vi "更新程序.vi"() -> ()   [LabVIEW 2016, in "自动更新.lvlib"]
uses:
  <vilib>/FTP/NI_FTP.lvlib
panel:
  out "updateconfiguration":T1
  out "软件版本 2":string caption="目标软件版本"
  out "软件版本":string caption="当前软件版本"
  out "下载的文件名":string
  out "目标文件夹名":string
  out "端口号":i32
  out "IP地址":string
  out "步骤":string
  out "枚举":T2(ring)
  in  "目标路径（使用对话框）":path
  out "下载保存目录":path
  out "更新进度":u8(slide) scale=0.0..100.0
  # "1.先下载更新-------2.关闭主应用-------3.替换应用--------4.打开主应用-----------5.关闭本程序"
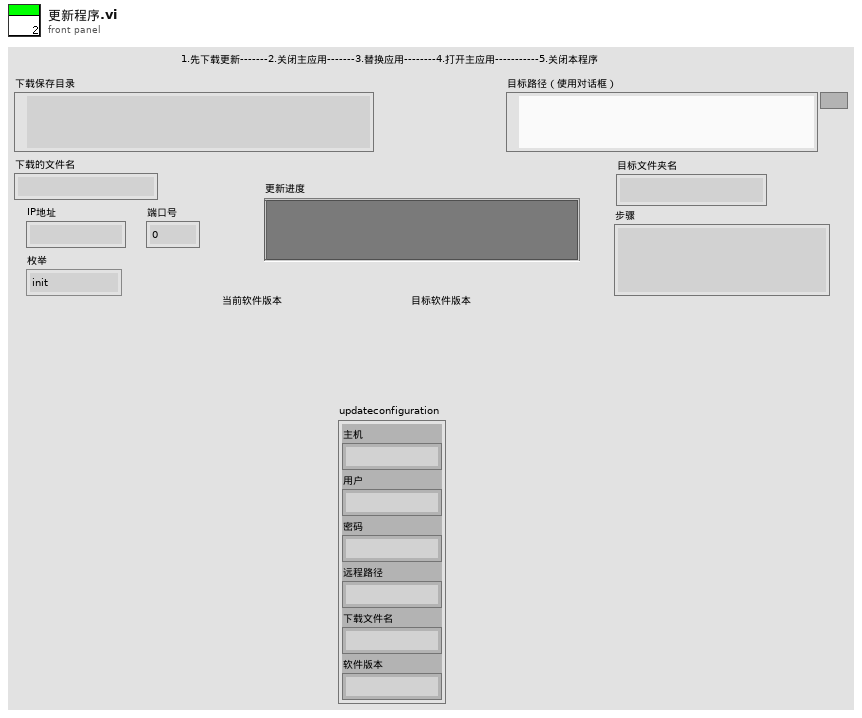
[diagram p1: front panel]
types:
  T1 = cluster{"主机":string, "用户":string, "密码":string, "远程路径":string, "下载文件名":string, "软件版本":string}
  T2 = enum16{"init", "download", "close", "replace", "open", "over"}
  T3 = enum16{"open", "replace", "create", "open or create", "replace or create", "replace or create with confirmation"}
  T4 = cluster{"网络灯":bool, "接收中":bool, "已接收百分比":u8, "接收成功次数":dbl, "当前步骤":enum16{"init", "receivehead", "receivecontent", "receivesuccess", "over"}, "文件名":string, "error out":errorcluster}
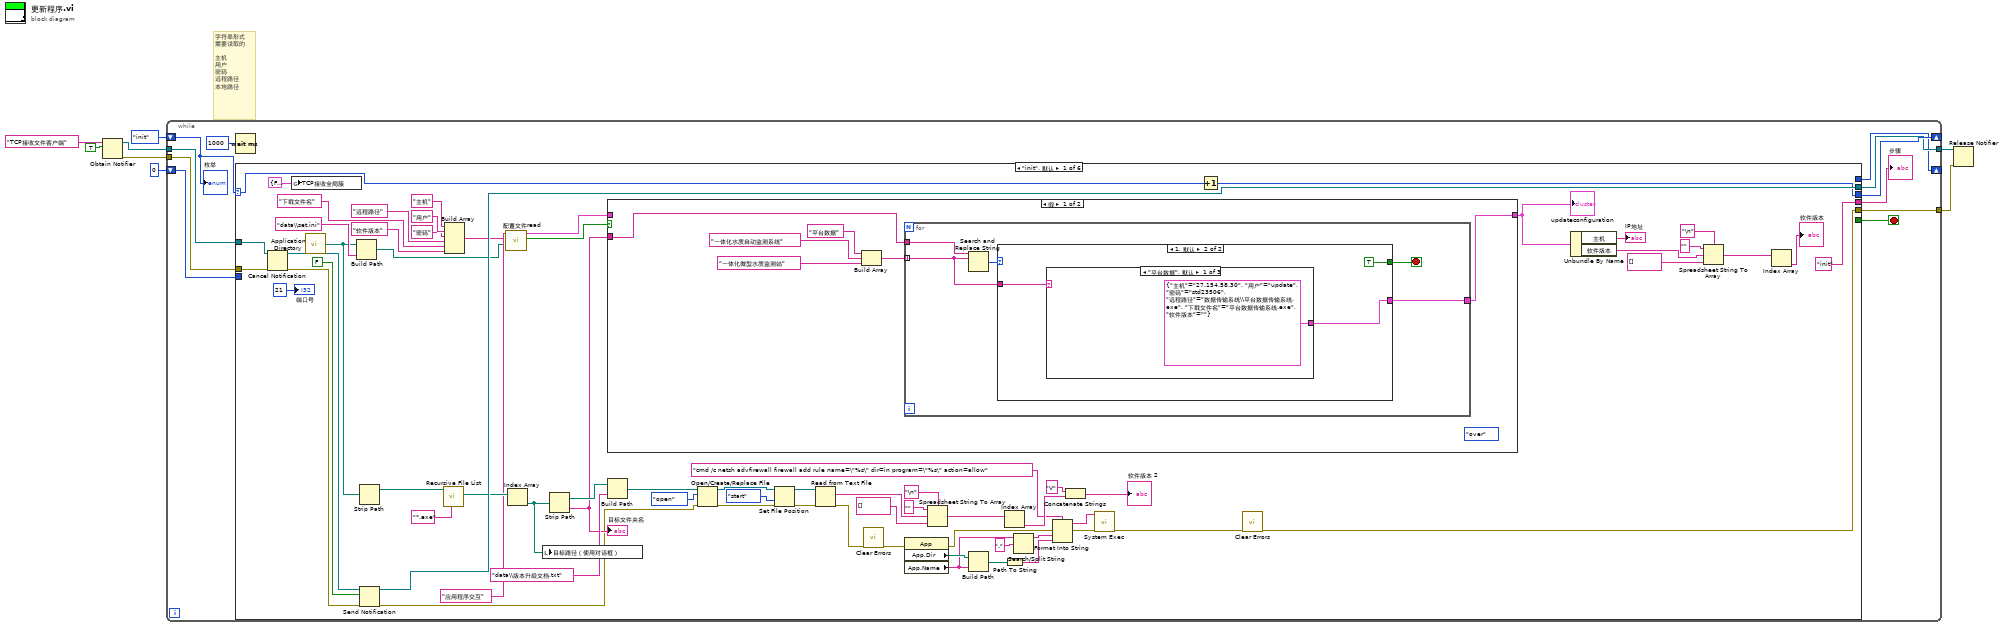
[diagram p0: block diagram]
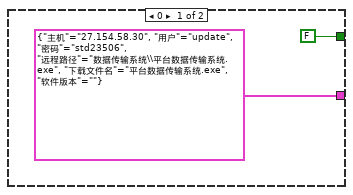
[diagram p2: hidden frame]
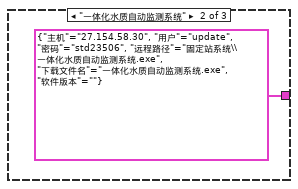
[diagram p3: hidden frame]
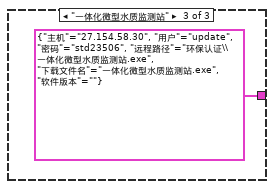
[diagram p4: hidden frame]
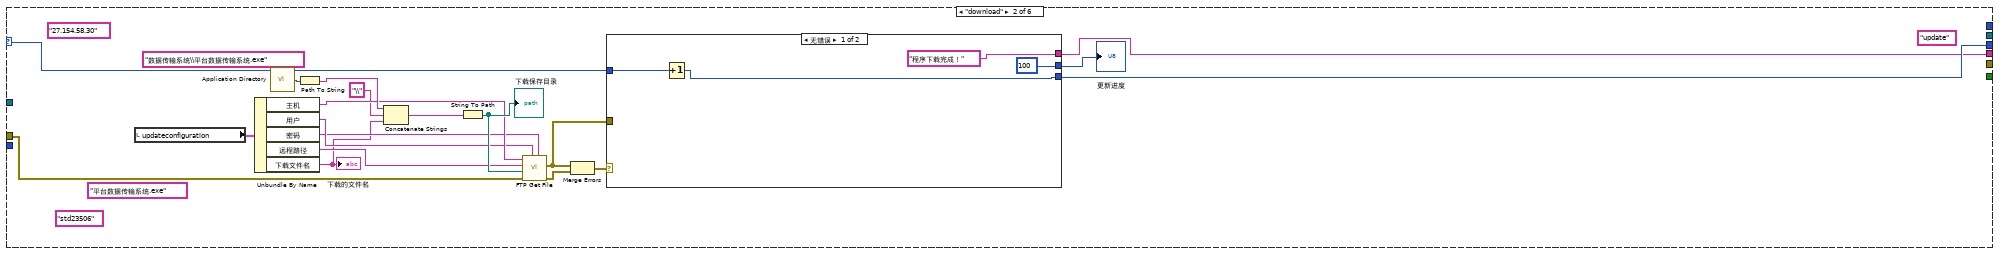
[diagram p6: hidden frame]
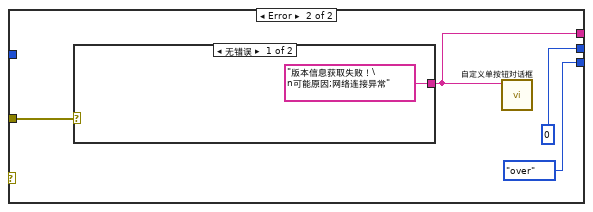
[diagram p7: hidden frame]
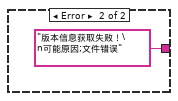
[diagram p8: hidden frame]
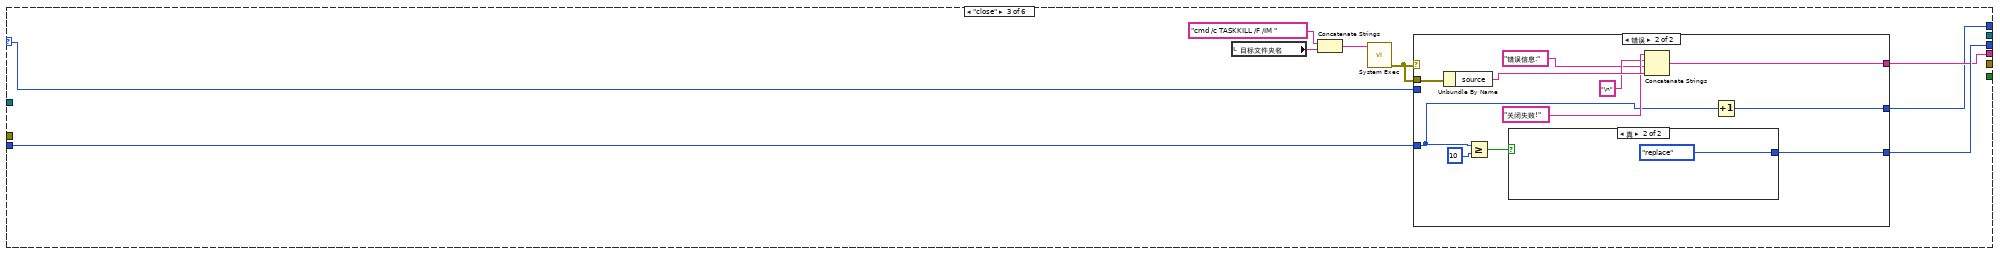
[diagram p9: hidden frame]
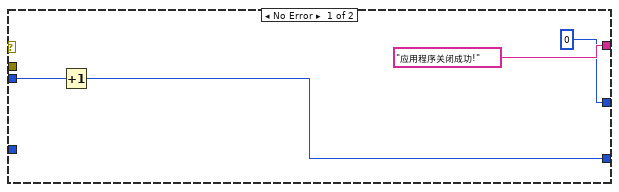
[diagram p10: hidden frame]
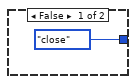
[diagram p11: hidden frame]
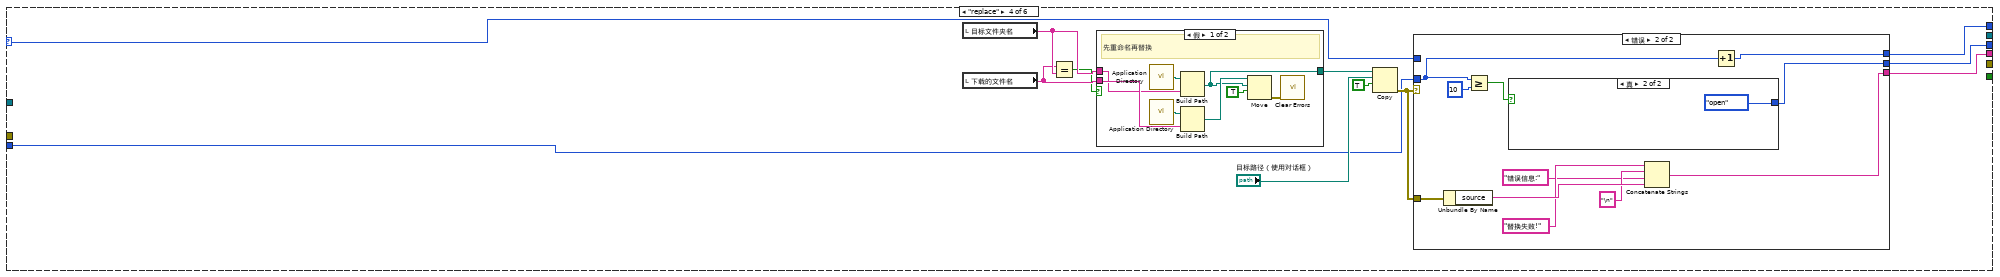
[diagram p12: hidden frame]
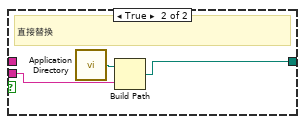
[diagram p13: hidden frame]
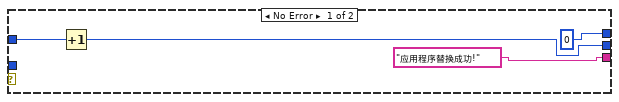
[diagram p14: hidden frame]
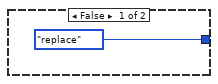
[diagram p15: hidden frame]
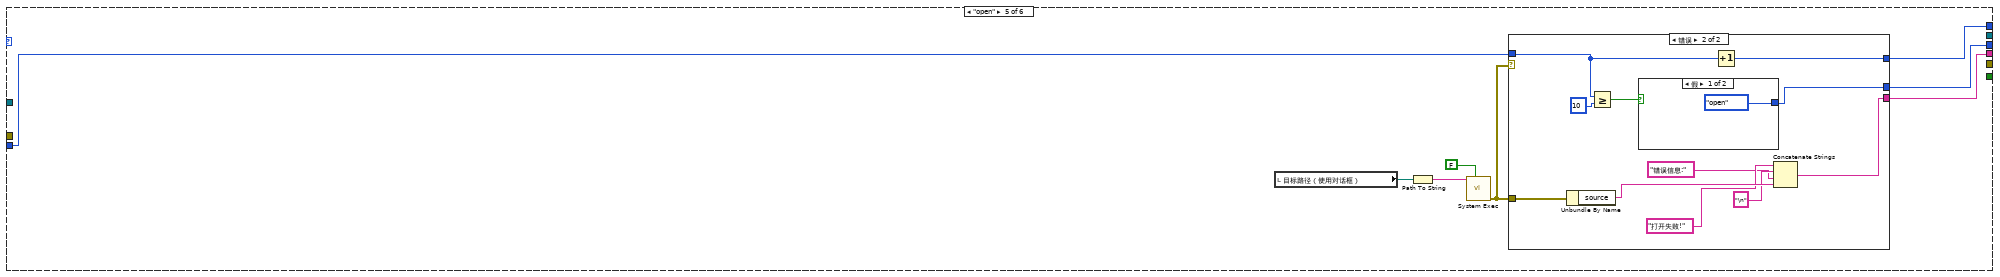
[diagram p16: hidden frame]
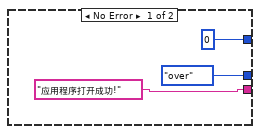
[diagram p17: hidden frame]
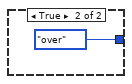
[diagram p18: hidden frame]
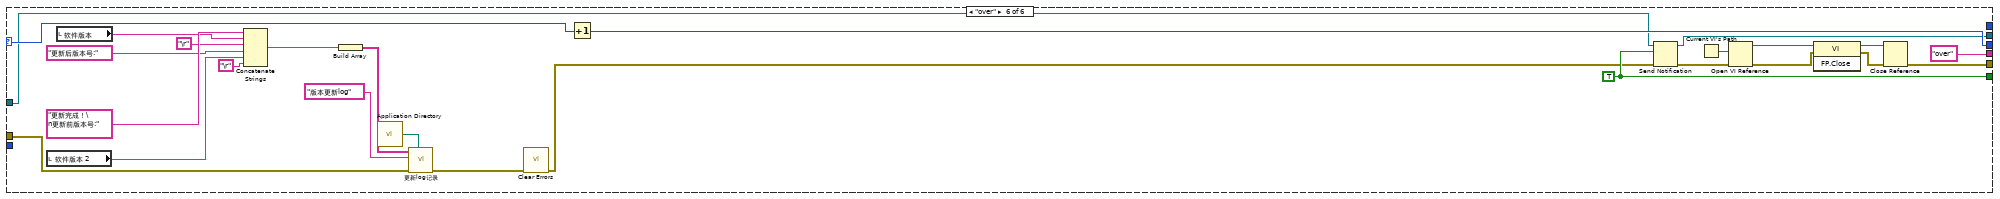
[diagram p19: hidden frame]
diagram:
  # "字符串形式\n需要读取的\n\n主机\n用户\n密码\n远程路径\n本地路径"
  n1 = Obtain Notifier(name (unnamed)="TCP接收文件客户端" ("名称（未命名）"), notification data type=TRUE) -> (notifier out=w5:refnum<notifier>, error out=w4:errorcluster)  [unwired: 2 in, 1 out]
  n2 = while {
    shift-right: [w18] -> _
    shift-left: T2."init" -> [w19]
    tunnel: w5 -> [w14]
    tunnel: w4 -> [w13]
    tunnel: [w12] -> w3
    tunnel: [w11] -> w2
    shift-right: [w9] -> _
    shift-left: u8 0 -> [w10]
    stop <- w17 stop-if-true
    n3 = Wait (ms)(milliseconds to wait=u32 1000 ("等待时间（毫秒）")) -> ()  [unwired: 1 out]
    n4 = case shown="\"init\", 默认" w19 {
      selector: w19 -> [w36 w122 w143 w175 _ w253]
      tunnel: [w35 w123 w142 w174 w207 w252] -> w18
      tunnel: [_ _ _ _ _ w248] -> w17
      tunnel: ["init" ("步骤") w120 w141 w173 w206 "over" ("步骤")] -> w15
      tunnel: w14 -> [w87 _ _ _ _ w250]
      tunnel: w13 -> [w86 w121 _ _ _ w240]
      tunnel: [w82 _ _ _ _ w249] -> w12
      tunnel: [w21 _ _ _ _ w232] -> w11
      tunnel: w10 -> [_ _ w139 w165 w204 _]
      tunnel: [_ _ w138 w164 w205 _] -> w9
      frame "init", Default {
        n5 = Cancel Notification(0:w87, 3:w86) -> (8:w85:refnum<notifier>, 11:w83:errorcluster)  [unwired: 1 out]
        n6 = global write "全局变量1.vi" "TCP接收全局簇"(T4 {"网络灯"=FALSE, "接收中"=FALSE, "已接收百分比"=0, "接收成功次数"=0.0, "当前步骤"=enum."init", "文件名"="", "error out"={"status"=FALSE, "code"=0, "source"=""}} ("TCP接收全局簇")) -> ()
        n7 = call <vilib>:"Application Directory.vi"() -> ("Application Directory"=w43:path)
        n8 = Build Path(base path=w43, name or relative path="data\\set.ini" ("名称或相对路径")) -> (appended path=w46:path)
        n9 = Strip Path(path=w43) -> (stripped path=w77:path)  [unwired: 1 out]
        n10 = Send Notification(notification=FALSE ("通知"), notifier=w85, error in (no error)=w83) -> (notifier out=w82:refnum<notifier>, error out=w22:errorcluster)
        n11 = call <vilib>:"Recursive File List.vi"("pattern"="*.exe", "Folder Path"=w77) -> ("All Files in Dir"=w79:path[])  [unwired: 5 in, 4 out]
        n12 = Build Array("主机" ("section"), "用户" ("section"), "密码" ("key"), "远程路径" ("key"), "下载文件名" ("key"), "软件版本" ("key")) -> (w50:string[])
        n13 = call "配置文件read.vi"("configuration file path"=w46, "键数组"=w50, "段"="应用程序交互" ("section")) -> ("section exists?"=w52:bool, "updateconfiguration"=w53:T1)  [unwired: 6 in, 1 out]
        n14 = Index Array(array=w79) -> (element=w80:path)  [unwired: 1 in]
        n15 = local write "目标路径（使用对话框）"(w80) -> ()
        n16 = Strip Path(path=w80) -> (stripped path=w54:path, name=w37:string)
        "目标文件夹名" <- w37
        n17 = case shown="假" w52 {
          tunnel: w53 -> [_ w108]
          tunnel: [w89 w108] -> w45
          tunnel: w37 -> [w90 _]
          frame False {
            (unwired) T2."over"
            n18 = Build Array("平台数据" ("搜索字符串"), "一体化水质自动监测系统" ("搜索字符串"), "一体化微型水质监测站" ("搜索字符串")) -> (w91:string[])
            n19 = for {
              tunnel: w91 -> [w96] mode=indexing
              tunnel: w90 -> [w97]
              tunnel: [w95] -> w89
              stop <- w98 stop-if-true
              n20 = Search and Replace String(input string=w97, search string=w96) -> (number of replacements=w99:i32)  [unwired: 6 in, 3 out]
              n21 = case shown="1, 默认" w99 {
                tunnel: [FALSE TRUE] -> w98
                tunnel: w96 -> [_ w103]
                tunnel: [T1 {"主机"="27.154.58.30", "用户"="update", "密码"="std23506", "远程路径"="数据传输系统\\平台数据传输系统.exe", "下载文件名"="平台数据传输系统.exe", "软件版本"=""} ("updateconfiguration") w102] -> w95
                frame 0 {
                }
                frame 1, Default {
                  n22 = case shown="\"平台数据\", 默认" w103 {
                    tunnel: [T1 {"主机"="27.154.58.30", "用户"="update", "密码"="std23506", "远程路径"="数据传输系统\\平台数据传输系统.exe", "下载文件名"="平台数据传输系统.exe", "软件版本"=""} ("updateconfiguration") T1 {"主机"="27.154.58.30", "用户"="update", "密码"="std23506", "远程路径"="固定站系统\\一体化水质自动监测系统.exe", "下载文件名"="一体化水质自动监测系统.exe", "软件版本"=""} ("updateconfiguration") T1 {"主机"="27.154.58.30", "用户"="update", "密码"="std23506", "远程路径"="环保认证\\一体化微型水质监测站.exe", "下载文件名"="一体化微型水质监测站.exe", "软件版本"=""} ("updateconfiguration")] -> w102
                    frame "平台数据", Default {
                    }
                    frame "一体化水质自动监测系统" {
                    }
                    frame "一体化微型水质监测站" {
                    }
                  }
                }
              }
            }
          }
          frame True {
          }
        }
        "updateconfiguration" <- w45
        n23 = Build Path(base path=w54, name or relative path="data\\版本升级文档.txt" ("名称或相对路径")) -> (appended path=w62:path)
        n24 = Open/Create/Replace File(file path (use dialog)=w62, error in=w22, operation (0:open)=T3."open" ("操作(0:open)")) -> (refnum out=w57:refnum<file>, error out=w58:errorcluster)  [unwired: 3 in, 1 out]
        n25 = Set File Position(refnum=w57, from (0:start)=enum16{"start", "end", "current"}."start" ("自（0:起始）"), error in=w58) -> (refnum out=w61:refnum<file>, error out=w59:errorcluster)  [unwired: 1 in]
        n26 = Read from Text File(file (use dialog)=w61, error in=w59) -> (text=w69:string, error out=w26:errorcluster)  [unwired: 2 in, 2 out]
        n27 = call <vilib>:"Clear Errors.vi"("error in (no error)"=w26) -> ("error out"=w20:errorcluster)  [unwired: 5 in, 1 out]
        n28 = property class="App"(error in=w20) -> (error out=w25:errorcluster, "App.Dir"=w34:path, "App.Name"=w29:string)  [unwired: 1 in, 1 out]
        n29 = Spreadsheet String To Array(delimiter (Tab)="\n" ("分隔符(Tab)"), format string="" ("格式字符串"), spreadsheet string=w69, array type (2D Dbl)=string[] []) -> (array=w66:string[])
        n30 = Build Path(base path=w34, name or relative path=w29) -> (appended path=w33:path)
        n31 = Index Array(array=w66) -> (element=w67:string)  [unwired: 1 in]
        n32 = Path To String(path=w33) -> (string=w31:string)
        n33 = Search/Split String(string=w29, search string/char (-)="." ("搜索字符串/字符(-)")) -> (substring before match=w28:string)  [unwired: 1 in, 2 out]
        n34 = Format Into String(format string="cmd /c netsh advfirewall firewall add rule name=\"%s\" dir=in program=\"%s\" action=allow" ("command line"), error in=w25, w28, w31) -> (resulting string=w27:string, error out=w24:errorcluster)  [unwired: 1 in]
        n35 = Concatenate Strings("V" ("字符串"), w67) -> (→"软件版本 2":string)
        n36 = call <vilib>:"System Exec.vi"("error in (no error)"=w24, "command line"=w27) -> ("error out"=w23:errorcluster)  [unwired: 6 in, 3 out]
        n37 = Increment(x=w36) -> (x+1=w35:T2)
        n38 = call <vilib>:"Clear Errors.vi"("error in (no error)"=w23) -> ("error out"=w21:errorcluster)  [unwired: 5 in, 1 out]
        n39 = Unbundle By Name(w45) -> ("主机"=→"IP地址":string, "软件版本"=w38:string)
        n40 = Spreadsheet String To Array(delimiter (Tab)="\n" ("分隔符(Tab)"), format string="" ("格式字符串"), spreadsheet string=w38, array type (2D Dbl)=string[] []) -> (array=w72:string[])
        n41 = Index Array(array=w72) -> (element=→"软件版本":string)  [unwired: 1 in]
        "端口号" <- 21 ("端口号")
      }
      frame "download" {
        (unwired) "平台数据传输系统.exe" ("字符串")
        (unwired) "std23506" ("password")
        (unwired) "update" ("user")
        (unwired) "数据传输系统\\平台数据传输系统.exe" ("remote path")
        (unwired) "27.154.58.30" ("host")
        n42 = local read "updateconfiguration"() -> (w115:T1)
        n43 = Unbundle By Name(w115) -> ("主机"=w114:string, "用户"=w113:string, "密码"=w112:string, "远程路径"=w111:string, "下载文件名"=w109:string)
        "下载的文件名" <- w109
        n44 = call <vilib>:"Application Directory.vi"() -> ("Application Directory"=w119:path)
        n45 = Path To String(path=w119) -> (string=w118:string)
        n46 = Concatenate Strings(w118, "\\" ("字符串"), w109) -> (w117:string)
        n47 = String To Path(string=w117) -> (path=w116:path)
        "下载保存目录" <- w116
        n48 = call <vilib>:"FTP Get File.vi"("password"=w112, "user"=w113, "error in (no error)"=w121, "local path"=w116, "remote path"=w111, "host"=w114) -> ("error out"=w127:errorcluster, "file error"=w126:errorcluster)  [unwired: 4 in]
        n49 = Merge Errors(w126, w127) -> (w125:errorcluster)
        n50 = case shown="无错误" w125 {
          tunnel: w126 -> [_ w135]
          tunnel: [u8 100 ("y") u8 0 ("y")] -> w124
          tunnel: [w130 T2."over"] -> w123
          tunnel: w122 -> [w129 _]
          tunnel: ["程序下载完成！" w132] -> w120
          frame No Error {
            n51 = Increment(x=w129) -> (x+1=w130:T2)
          }
          frame Error {
            n52 = case shown="无错误" w135 {
              tunnel: ["版本信息获取失败！\n可能原因;网络连接异常" "版本信息获取失败！\n可能原因;文件错误"] -> w132
              frame No Error {
              }
              frame Error {
              }
            }
            n53 = call "自定义单按钮对话框.vi"("消息"=w132) -> ()  [unwired: 11 in]
          }
        }
        "更新进度" <- w124
      }
      frame "close" {
        n54 = local read "目标文件夹名"() -> (w140:string)
        n55 = Concatenate Strings("cmd /c TASKKILL /F /IM " ("command line"), w140) -> (w144:string)
        n56 = call <vilib>:"System Exec.vi"("command line"=w144) -> ("error out"=w146:errorcluster)  [unwired: 7 in, 3 out]
        n57 = case shown="错误" w146 {
          tunnel: [w148 w155] -> w142
          tunnel: w146 -> [_ w161]
          tunnel: ["应用程序关闭成功!" ("步骤") w156] -> w141
          tunnel: w143 -> [w149 _]
          tunnel: w139 -> [_ w151]
          tunnel: [u8 0 w153] -> w138
          frame No Error {
            n58 = Increment(x=w149) -> (x+1=w148:T2)
          }
          frame Error {
            n59 = Unbundle By Name(w161) -> ("source"=w160:string)
            n60 = Greater Or Equal?(x=w151, y=u8 10) -> (x >= y?=w152:bool)
            n61 = case shown="真" w152 {
              tunnel: [T2."close" T2."replace"] -> w155
              frame False {
              }
              frame True {
              }
            }
            n62 = Concatenate Strings("关闭失败!" ("消息"), "\n" ("字符串"), "错误信息:" ("字符串"), w160) -> (w156:string)
            n63 = Increment(x=w151) -> (x+1=w153:u8)
          }
        }
      }
      frame "replace" {
        n64 = local read "目标文件夹名"() -> (w169:string)
        n65 = local read "下载的文件名"() -> (w168:string)
        n66 = Equal?(x=w168, y=w169) -> (x = y?=w167:bool)
        n67 = case shown="假" w167 {
          tunnel: w168 -> [w180 w185]
          tunnel: w169 -> [w179 _]
          tunnel: [w178 w184] -> w172
          frame False {
            # "先重命名再替换"
            n68 = call <vilib>:"Application Directory.vi"() -> ("Application Directory"=w182:path)
            n69 = call <vilib>:"Application Directory.vi"() -> ("Application Directory"=w181:path)
            n70 = Build Path(base path=w182, name or relative path=w179) -> (appended path=w178:path)
            n71 = Build Path(base path=w181, name or relative path=w180) -> (appended path=w183:path)
            n72 = Move(source path=w183, 9:TRUE ("覆盖(F)"), 10:w178) -> (error out=w176:errorcluster)  [unwired: 2 in, 2 out]
            n73 = call <vilib>:"Clear Errors.vi"("error in (no error)"=w176) -> ()  [unwired: 5 in, 2 out]
          }
          frame True {
            # "直接替换"
            n74 = call <vilib>:"Application Directory.vi"() -> ("Application Directory"=w186:path)
            n75 = Build Path(base path=w186, name or relative path=w185) -> (appended path=w184:path)
          }
        }
        n76 = Copy(9:TRUE ("覆盖(F)"), 10:"目标路径（使用对话框）", 11:w172) -> (0:w166:errorcluster)  [unwired: 2 in, 2 out]
        n77 = case shown="错误" w166 {
          tunnel: [w188 w195] -> w174
          tunnel: w166 -> [_ w201]
          tunnel: ["应用程序替换成功!" ("步骤") w196] -> w173
          tunnel: w175 -> [w189 _]
          tunnel: w165 -> [_ w193]
          tunnel: [u8 0 w191] -> w164
          frame No Error {
            n78 = Increment(x=w189) -> (x+1=w188:T2)
          }
          frame Error {
            n79 = Unbundle By Name(w201) -> ("source"=w200:string)
            n80 = Greater Or Equal?(x=w193, y=u8 10) -> (x >= y?=w192:bool)
            n81 = case shown="真" w192 {
              tunnel: [T2."replace" T2."open"] -> w195
              frame False {
              }
              frame True {
              }
            }
            n82 = Concatenate Strings("替换失败!" ("消息"), "\n" ("字符串"), "错误信息:" ("字符串"), w200) -> (w196:string)
            n83 = Increment(x=w193) -> (x+1=w191:u8)
          }
        }
      }
      frame "open" {
        n84 = local read "目标路径（使用对话框）"() -> (w208:path)
        n85 = Path To String(path=w208) -> (string=w211:string)
        n86 = call <vilib>:"System Exec.vi"("wait until completion? (T)"=FALSE, "command line"=w211) -> ("error out"=w209:errorcluster)  [unwired: 6 in, 3 out]
        n87 = case shown="错误" w209 {
          tunnel: [T2."over" w219] -> w207
          tunnel: w209 -> [_ w225]
          tunnel: ["应用程序打开成功!" ("步骤") w220] -> w206
          tunnel: w204 -> [_ w217]
          tunnel: [u8 0 w215] -> w205
          frame No Error {
          }
          frame Error {
            n88 = Unbundle By Name(w225) -> ("source"=w224:string)
            n89 = Greater Or Equal?(x=w217, y=u8 10) -> (x >= y?=w216:bool)
            n90 = case shown="假" w216 {
              tunnel: [T2."open" T2."over"] -> w219
              frame False {
              }
              frame True {
              }
            }
            n91 = Increment(x=w217) -> (x+1=w215:u8)
            n92 = Concatenate Strings("打开失败!" ("消息"), "\n" ("字符串"), "错误信息:" ("字符串"), w224) -> (w220:string)
          }
        }
      }
      frame "over" {
        w248 = TRUE
        n93 = local read "软件版本 2"() -> (w229:string)
        n94 = local read "软件版本"() -> (w231:string)
        n95 = Concatenate Strings("更新完成！\n更新前版本号:" ("字符串"), w231, "\r", "更新后版本号:", w229, "\r") -> (w246:string)
        n96 = Build Array(w246) -> (w245:string[])
        n97 = call <vilib>:"Application Directory.vi"() -> ("Application Directory"=w243:path)
        n98 = call "更新log记录.vi"("路径"=w243, "错误输入（无错误）"=w240, "logname"="版本更新log", "数组"=w245) -> ("错误输出"=w241:errorcluster)  [unwired: 7 in]
        n99 = call <vilib>:"Clear Errors.vi"("error in (no error)"=w241) -> ("error out"=w239:errorcluster)  [unwired: 5 in, 1 out]
        n100 = Increment(x=w253) -> (x+1=w252:T2)
        n101 = Send Notification(notification=w248, notifier=w250, error in (no error)=w239) -> (notifier out=w249:refnum<notifier>, error out=w235:errorcluster)
        n102 = Current VI's Path() -> (path=w237:path)
        n103 = Open VI Reference(vi path=w237, error in (no error)=w235) -> (vi reference=w236:refnum<vi>, error out=w238:errorcluster)  [unwired: 4 in]
        n104 = invoke class="VI" method="FP.Close"(reference=w236, error in=w238) -> (reference out=w233:refnum<vi>, error out=w234:errorcluster)  [unwired: 1 in, 1 out]
        n105 = Close Reference(reference=w233, error in (no error)=w234) -> (error out=w232:errorcluster)
      }
    }
    "步骤" <- w15
    "枚举" <- w19
  }
  n106 = Release Notifier(notifier=w3, error in (no error)=w2) -> ()  [unwired: 1 in, 3 out]
